vi "TTA_Execute_List.vi"(0 "Section List":T3 caption="RFIC List", 1 "Test Status Refnum":refnum<vi>, 2 "Complete Settings Cluster":T2, 5 "TTA FP\nRFIC Refnum In":refnum<vi>, 7 "Tile Section":enum16{"RFIC", "Tx", "Rx"}(ring), 9 "Channel Cluster":cluster{"Channel 1":bool, "Channel 2":bool}, 11 "error in":errorcluster, 12 "Instrument Cluster In":T1) -> (15 "error out":errorcluster)   [LabVIEW 2016]
uses:
  TTA_Controls/TTA_Control_RFIC_List.ctl
  TTA_Controls/TTA_Control_Complete_Settings_Cluster.ctl
  TTA_Controls/TTA_Control_Instrument_Cluster.ctl
  TTA_Globals/Test_Environment.vi
  TTA_Globals/TTA_Global_Complete_Settings.vi
panel:
  out "Instrument Cluster Out":T1
  in  "Complete":string="Complete"
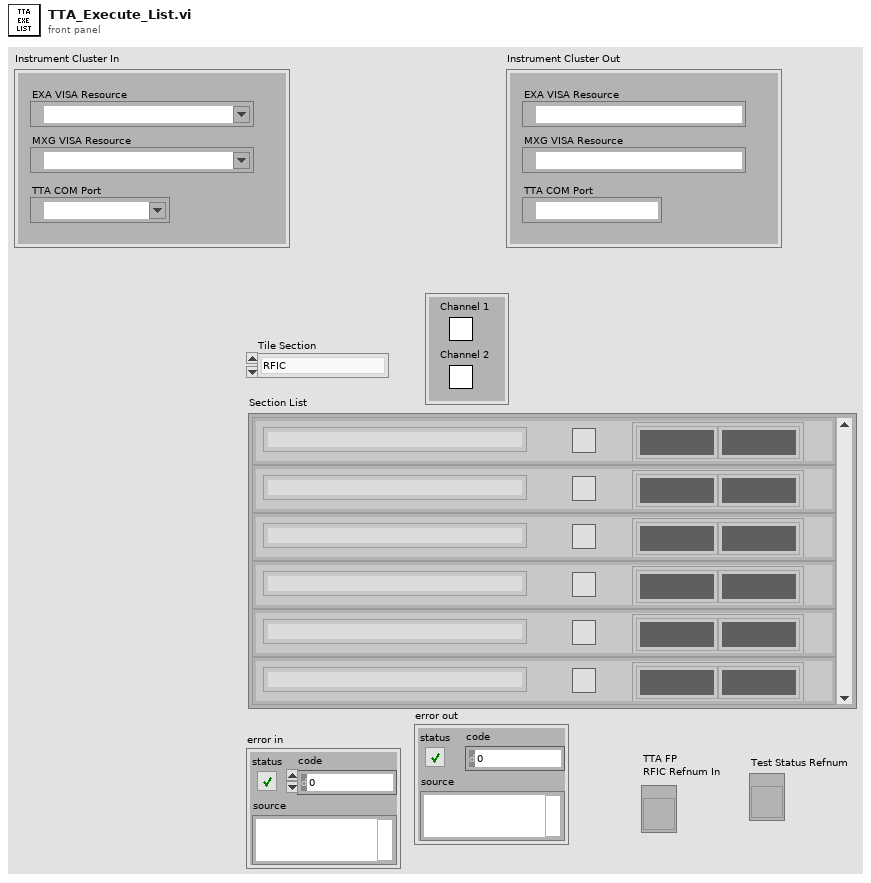
[diagram p1: front panel]
types:
  T1 = typedef "TTA_Control_Instrument_Cluster.ctl" = cluster{"EXA VISA Resource":refnum<visa-resource-name>, "MXG VISA Resource":refnum<visa-resource-name>, "TTA COM Port":refnum<visa-resource-name>}
  T2 = typedef "TTA_Control_Complete_Settings_Cluster.ctl" = cluster{"Brief Cluster":cluster{"STM Firmware File":string, "STM Firmware Address":string, "Required SW Version":string, "Template Used":string}, "Instrument Setting Cluster":cluster{"BDSFreq":dbl, "BDS Amp":dbl, "TxRFCal_Freq":dbl, "TxRFCal_Amp":dbl, "RxRFCal_Freq":dbl, "RxRFCal_Freq":dbl, "TxIF_Freq":dbl, "TxIF_Amp":dbl, "Tx_Output_Power_Signal_Freq":dbl, "Tx_ACPR_Signal_Freq":dbl, "Rx_RF_Freq":dbl, "Rx_RF_Amp":dbl, "Rx_Output_Power_Signal_Freq":dbl, "Rx_Output_Power_Sense_Freq":dbl}, "PAL Calibration\nInputs Cluster":cluster{"Amplitude Range\nMax(dBm)":dbl, "Amplitude Range\nMin(dBm)":dbl, "Amplitude Least\nCriteria (dBm)":dbl, "Frequency 1":dbl, "Frequency 2":dbl, "Frequency 3":dbl, "CAL Amplitude\nDecrement (dB)":dbl, "CAL Amplitude\nIncrement(dB)":dbl, "DownloadFile":string}, "TxOffset Cal Cluster":cluster{"Tx1 Offset (dB)":dbl, "Tx2 Offset (dB)":dbl, "Tx3 Offset (dB)":dbl, "Tx4 Offset (dB)":dbl, "Total RF Tx Loss (dB)":dbl}, "RxOffset Cal Cluster":cluster{"Rx1 Offset (dB)":dbl, "Rx2 Offset (dB)":dbl, "Rx3 Offset (dB)":dbl, "Rx4 Offset (dB)":dbl, "Total RF Rx Loss (dB)":dbl}, "TX Output Power Settings Cluster":cluster{"Frequency Sweep (MHz)":dbl[], "Sig Gen \nPower (dBm)":dbl, "Span (kHz)":dbl, "RBW (Hz)":dbl, "Ref Level (dBm)":dbl, "Low Power \nLimit":dbl, "High Power \nLimit":dbl, "DigAtt Max":dbl, "DigAtt Min":dbl}, "Tx ACPR Settings Cluster":cluster{"ACPR Filename":string, "Sampling Rate":dbl, "Power (dBm)":dbl, "IF Frequency Sweep (MHz)":dbl[], "State Name":string, "Mechanical\nAttenuation":dbl, "RefLevel Offset":dbl, "Amplitude Range\nMax (dBm)":dbl, "Amplitude Range\nMin (dBm)":dbl, "Cal Amp \nIncrement (dB)":dbl, "Cal Amp\nDecrement (dB)":dbl}, "Power Cal Cluster":cluster{"Power List (dBm)":dbl[], "Frequency (MHz)":dbl[], "Cal Decrement (dB)":dbl, "Cal Increment (dB)":dbl}, "Rx Received Power Settings Cluster":cluster{"Frequency Sweep (MHz)":dbl[], "Power (dBm)":dbl, "Span (kHz)":dbl, "RBW (Hz)":dbl, "Ref Level":dbl, "Low Power \nLimit (dBm)":dbl, "High Power\nLimit (dBm)":dbl}, "Tx Output Power Criteria Cluster":cluster{"CH1-TX1 \nMin":dbl, "CH1-TX1\nMax":dbl, "CH1-TXx3\nMin ":dbl, "CH1-TXx3\nMax":dbl, "CH2-TX1\nMin":dbl, "CH2-TX1\nMax":dbl, "CH2-TXx3\nMin":dbl, "CH2-TXx3\nMax":dbl}, "Tx ACPR Criteria Cluster":cluster{"Min Inband":dbl, "Max Close Outband":dbl, "Max Far Outband":dbl}, "Rx Output Power Criteria Cluster":cluster{"CH1-RX1 \nMin":dbl, "CH1-RX1 \nMax":dbl, "CH1-RXx3 \nMin":dbl, "CH1-RXx3\nMax":dbl, "CH2-RX1\nMin":dbl, "CH2-RX1\nMax":dbl, "CH2-RXx3\nMin":dbl, "CH2-RXx3\nMax":dbl}}
  T3 = typedef "TTA_Control_RFIC_List.ctl" = cluster{"Enable":bool, "Test Description":string, "Status Array":u16[]}[]
  T4 = cluster{"Enable":bool, "Test Description":string, "Status Array":u16[]}
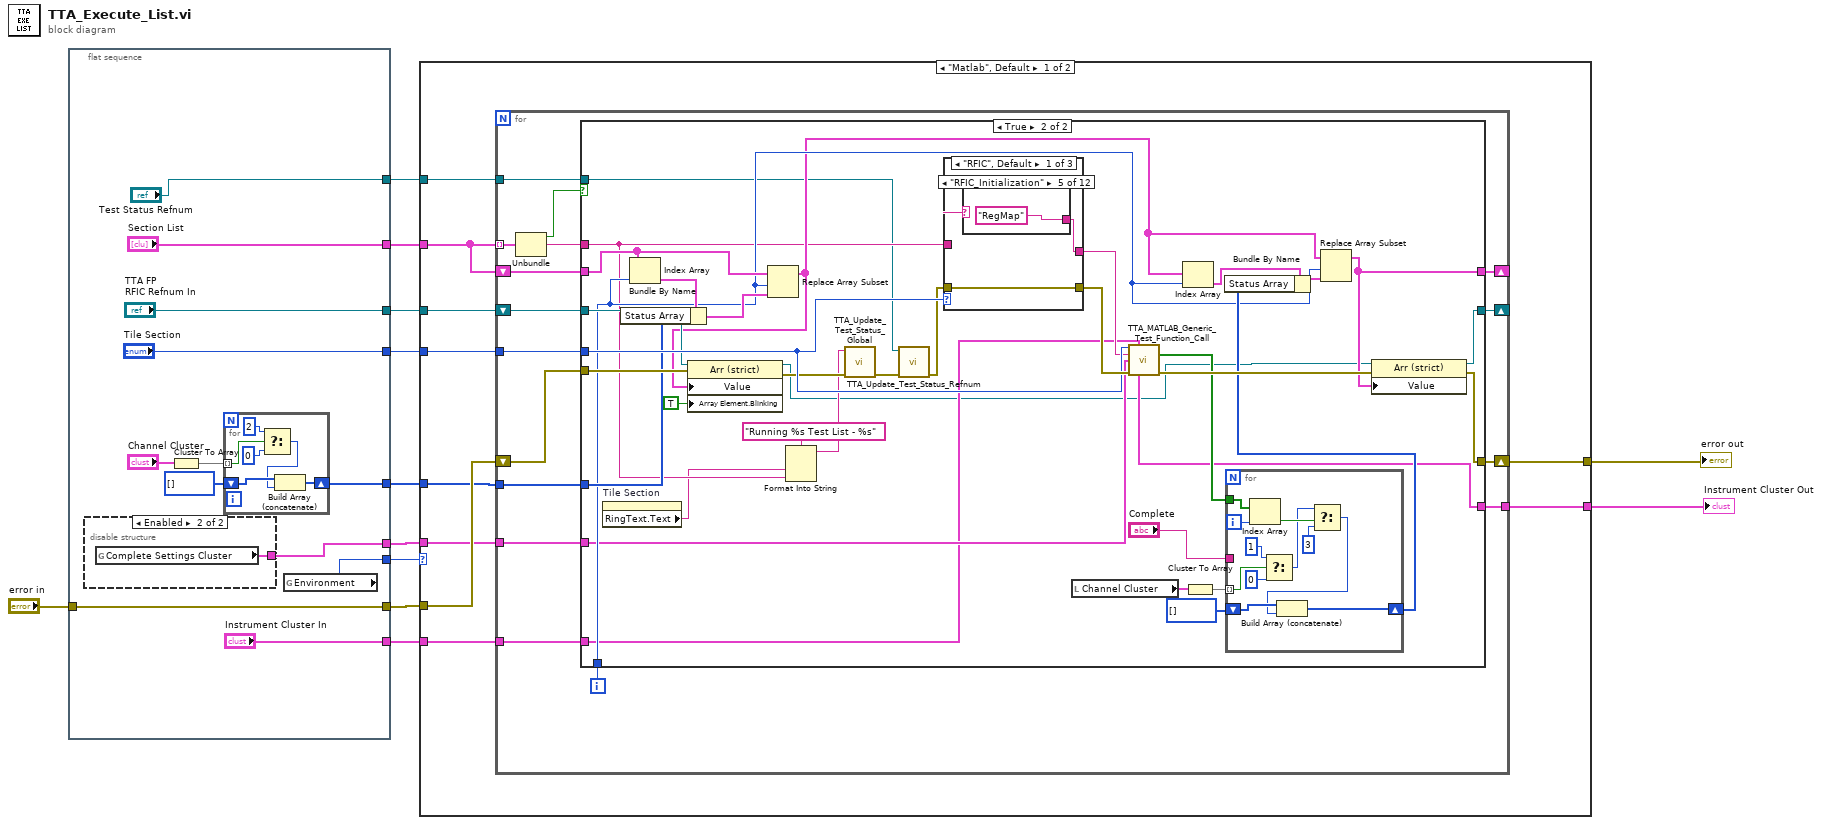
[diagram p0: block diagram]
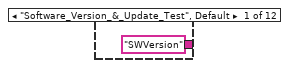
[diagram p3: hidden frame]
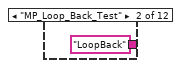
[diagram p4: hidden frame]
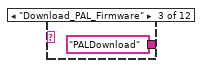
[diagram p5: hidden frame]
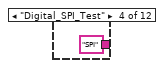
[diagram p6: hidden frame]
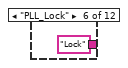
[diagram p7: hidden frame]
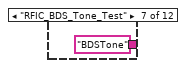
[diagram p8: hidden frame]
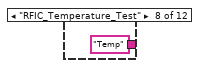
[diagram p9: hidden frame]
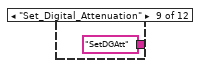
[diagram p10: hidden frame]
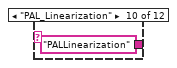
[diagram p11: hidden frame]
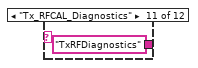
[diagram p12: hidden frame]
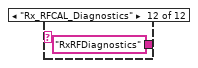
[diagram p13: hidden frame]
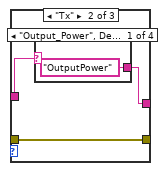
[diagram p14: hidden frame]
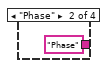
[diagram p15: hidden frame]
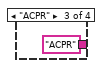
[diagram p16: hidden frame]
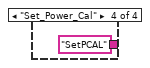
[diagram p17: hidden frame]
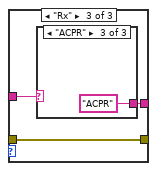
[diagram p18: hidden frame]
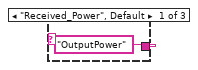
[diagram p19: hidden frame]
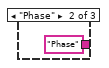
[diagram p20: hidden frame]
diagram:
  n1 = flat-sequence {
    tunnel: "error in" -> [w24]
    tunnel: [w24] -> w11
    tunnel: ["Section List"] -> w7
    tunnel: ["Tile Section"] -> w9
    tunnel: ["TTA FP\nRFIC Refnum In"] -> w8
    tunnel: [w18] -> w6
    tunnel: [w17] -> w5
    tunnel: ["Test Status Refnum"] -> w4
    tunnel: [w15] -> w3
    tunnel: ["Instrument Cluster In"] -> w2
    frame #0 {
      n2 = disable-structure shown="Enabled" {
        disable-tunnel: ["Complete Settings Cluster" w26] -> w15
        frame Disabled {
        }
        frame Enabled {
          n3 = global read "TTA_Global_Complete_Settings.vi" "Complete Settings Cluster"() -> (w26:T2)
        }
      }
      n4 = Cluster To Array(cluster="Channel Cluster") -> (array=w19:bool[])
      n5 = for {
        tunnel: w19 -> [w31] mode=indexing
        shift-right: [w32] -> w18
        shift-left: i32[] [] -> [w30]
        n6 = Select(t=2, s=w31, f=0) -> (s? t:f=w29:i32)
        n7 = Build Array (concatenate)(w30, w29) -> (w32:i32[])
      }
      n8 = global read "Test_Environment.vi" "Environment"() -> (w17:enum16{"Matlab", "LabVIEW"})
    }
  }
  n9 = case shown="\"Matlab\", Default" w5 {
    tunnel: w11 -> [w42 w139]
    tunnel: [w41 w139] -> w10
    tunnel: w9 -> [w40 _]
    tunnel: w8 -> [w39 _]
    tunnel: w7 -> [w38 _]
    tunnel: w6 -> [w37 _]
    tunnel: w4 -> [w36 _]
    tunnel: w3 -> [w35 _]
    tunnel: w2 -> [w34 w138]
    tunnel: [w33 w138] -> w1
    frame "Matlab", Default {
      n10 = for {
        shift-right: [w53] -> w41
        shift-left: w42 -> [w54]
        tunnel: w38 -> [w58] mode=indexing
        tunnel: w40 -> [w55]
        shift-right: [w49] -> _
        shift-left: w39 -> [w52]
        shift-right: [w47] -> _
        shift-left: w38 -> [w51]
        tunnel: w37 -> [w48]
        tunnel: w36 -> [w46]
        tunnel: w35 -> [w45]
        tunnel: w34 -> [w44]
        tunnel: [w43] -> w33
        i -> [w50]
        n11 = Unbundle(w58) -> ("Enable"=w57:bool, "Test Description"=w56:string)  [unwired: 1 out]
        n12 = case shown="True" w57 {
          tunnel: w56 -> [_ w72]
          tunnel: w55 -> [_ w97]
          tunnel: w54 -> [w62 w94]
          tunnel: [w62 w91] -> w53
          tunnel: w52 -> [w60 w93]
          tunnel: w51 -> [w61 w87]
          tunnel: w50 -> [_ w81]
          tunnel: [w60 w92] -> w49
          tunnel: w48 -> [_ w89]
          tunnel: [w61 w78] -> w47
          tunnel: w46 -> [_ w71]
          tunnel: w45 -> [_ w68]
          tunnel: w44 -> [w59 w67]
          tunnel: [w59 w66] -> w43
          frame False {
          }
          frame True {
            n13 = property on="Tile Section" class="Enum (strict)"() -> ("RingText.Text"=w69:string)  [unwired: 2 in, 2 out]
            n14 = Index Array(array=w87, index=w81) -> (element=w90:T4)
            n15 = Bundle By Name(cluster=w90, "Status Array"=w89) -> (w88:T4)
            n16 = Replace Array Subset(array=w87, new element=w88, index=w81) -> (w79:T3)
            n17 = property class="Arr (strict)"(reference=w93, error in=w94, "Value"=w79, "Array Element.Blinking"=TRUE) -> (reference out=w65:refnum<vi>, error out=w74:errorcluster)
            n18 = Format Into String(format string="Running %s Test List - %s", w69, w72) -> (resulting string=w70:string)  [unwired: 2 in, 1 out]
            n19 = call "TTA_Update_Test_Status_Global.vi"("error in"=w74, "Test Status"=w70) -> ("error out"=w75:errorcluster)  [unwired: 9 in]
            n20 = call "TTA_Update_Test_Status_Refnum.vi"("error in"=w75, "Test Status Refnum"=w71) -> ("error out"=w76:errorcluster)  [unwired: 9 in]
            n21 = case shown="\"RFIC\", Default" w97 {
              tunnel: w72 -> [w112 w127 w134]
              tunnel: [w111 w126 w133] -> w96
              tunnel: w76 -> [w110 w125 w132]
              tunnel: [w110 w125 w132] -> w98
              frame "RFIC", Default {
                n22 = case shown="\"RFIC_Initialization\"" w112 {
                  tunnel: ["SWVersion" "LoopBack" "PALDownload" "SPI" "RegMap" "Lock" "BDSTone" "Temp" "SetDGAtt" "PALLinearization" "TxRFDiagnostics" "RxRFDiagnostics"] -> w111
                  frame "Software_Version_&_Update_Test", Default {
                  }
                  frame "MP_Loop_Back_Test" {
                  }
                  frame "Download_PAL_Firmware" {
                  }
                  frame "Digital_SPI_Test" {
                  }
                  frame "RFIC_Initialization" {
                  }
                  frame "PLL_Lock" {
                  }
                  frame "RFIC_BDS_Tone_Test" {
                  }
                  frame "RFIC_Temperature_Test" {
                  }
                  frame "Set_Digital_Attenuation" {
                  }
                  frame "PAL_Linearization" {
                  }
                  frame "Tx_RFCAL_Diagnostics" {
                  }
                  frame "Rx_RFCAL_Diagnostics" {
                  }
                }
              }
              frame "Tx" {
                n23 = case shown="\"Output_Power\", Default" w127 {
                  tunnel: ["OutputPower" "Phase" "ACPR" "SetPCAL"] -> w126
                  frame "Output_Power", Default {
                  }
                  frame "Phase" {
                  }
                  frame "ACPR" {
                  }
                  frame "Set_Power_Cal" {
                  }
                }
              }
              frame "Rx" {
                n24 = case shown="\"ACPR\"" w134 {
                  tunnel: ["OutputPower" "Phase" "ACPR"] -> w133
                  frame "Received_Power", Default {
                  }
                  frame "Phase" {
                  }
                  frame "ACPR" {
                  }
                }
              }
            }
            n25 = local read "Channel Cluster"() -> (w86:cluster{"Channel 1":bool, "Channel 2":bool})
            n26 = call "TTA_MATLAB_Generic_Test_Function_Call.vi"("Tile Section"=w97, "Instrument Cluster In"=w67, "Sub-Function Name"=w96, "Complete Settings Cluster"=w68, "error in"=w98) -> ("SubTestSuccess"=w77:bool[], "Instrument Cluster Out"=w66:T1, "error out"=w95:errorcluster)  [unwired: 7 in, 1 out]
            n27 = Index Array(array=w79, index=w81) -> (element=w83:T4)
            n28 = Cluster To Array(cluster=w86) -> (array=w85:bool[])
            n29 = for {
              tunnel: w85 -> [w109] mode=indexing
              shift-right: [w107] -> w82
              shift-left: i32[] [] -> [w108]
              tunnel: "Complete" -> [_]
              tunnel: w77 -> [w106]
              i -> [w105]
              n30 = Index Array(array=w106, index=w105) -> (element=w104:bool)
              n31 = Select(t=1, s=w109, f=0) -> (s? t:f=w102:i32)
              n32 = Select(t=w102, s=w104, f=3) -> (s? t:f=w103:i32)
              n33 = Build Array (concatenate)(w108, w103) -> (w107:i32[])
            }
            n34 = Bundle By Name(cluster=w83, "Status Array"=w82) -> (w80:T4)
            n35 = Replace Array Subset(array=w79, new element=w80, index=w81) -> (w78:T3)
            n36 = property class="Arr (strict)"(reference=w65, error in=w95, "Value"=w78) -> (reference out=w92:refnum<vi>, error out=w91:errorcluster)
          }
        }
      }
    }
    frame "LabVIEW" {
    }
  }
  "error out" <- w10
  "Instrument Cluster Out" <- w1
